vi "WPI_PWMRefNum Registry Read Name.vi"(8 "error in (no error)":errorcluster, 11 "PWMDeviceRef":T1={"DeviceStatus"={"status"=FALSE, "code"=0, "source"=""}, "PWM Channel"=enum."PWM 1"}) -> (0 "error out":errorcluster, 2 "refnum name":string="My RobotDrive RefNum", 3 "PWMDeviceRef out":T1={"DeviceStatus"={"status"=FALSE, "code"=0, "source"=""}, "PWM Channel"=enum."PWM 1"})   [LabVIEW 2017]
doc: "Reads the name of a registered DevRef. You first must set the reference with the RefNum Registry Set VI. If the DevRef has not been registered, this VI returns an empty string."
uses:
  <vilib>/Rock Robotics/WPI/PWM/WPI_PWMDeviceRef.ctl
  <vilib>/Rock Robotics/SystemInterfaces/DIO/FPGA_DIOPWMChannel.ctl
  <vilib>/Rock Robotics/WPI/Utilities/Refnum Registry Operation.ctl
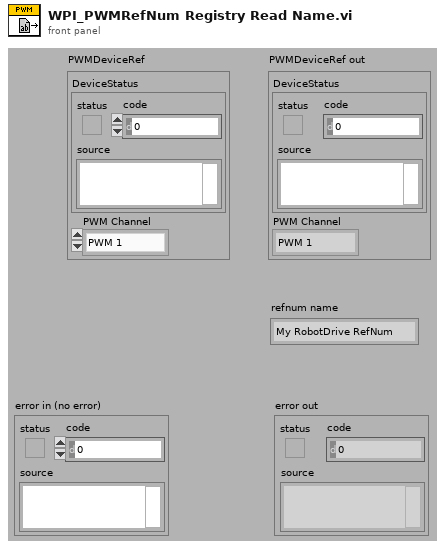
[diagram p1: front panel]
types:
  T1 = typedef "WPI_PWMDeviceRef.ctl" = cluster{"DeviceStatus":errorcluster, "PWM Channel":T2}
  T2 = typedef "FPGA_DIOPWMChannel.ctl" = enum8{"PWM 0", "PWM 1", "PWM 2", "PWM 3", "PWM 4", "PWM 5", "PWM 6", "PWM 7", "PWM 8", "PWM 9", "PWM MXP 0", "PWM MXP 1", "PWM MXP 2", "PWM MXP 3", "PWM MXP 4", "PWM MXP 5", "PWM MXP 6", "PWM MXP 7", "PWM MXP 8", "PWM MXP 9", "Invalid"}
  T3 = typedef "Refnum Registry Operation.ctl" = enum16{"set", "get", "delete", "get all names", "read name"}
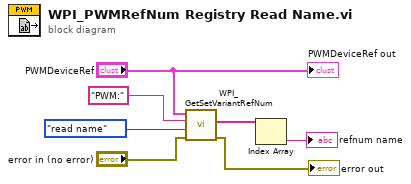
[diagram p0: block diagram]
diagram:
  n1 = call <vilib>:"WPI_GetSetVariantRefNum.vi"("error in (no error)"="error in (no error)", "Operation"=Refnum_Registry_Operation."read name" ("menu"), "refnum name"="PWM:", "DevRef"="PWMDeviceRef") -> ("error out"=→"error out":errorcluster, "names"=w3:string[])  [unwired: 5 in, 1 out]
  n2 = Index Array(array=w3) -> (element=→"refnum name":string)  [unwired: 1 in]
  "PWMDeviceRef out" <- "PWMDeviceRef"
